vi "Flatten Value.vi"(8 "Error In":errorcluster, 11 "Path Array In":refnum<class "1D Path.lvclass">) -> (0 "Error Out":errorcluster, 1 "Value":string, 3 "Path Array Out":refnum<class "1D Path.lvclass">)   [LabVIEW 2017, in "Tree API.lvlib" / "1D Path.lvclass"]
uses:
  1D Path.lvclass
  Tree Manager/Tree.lvclass
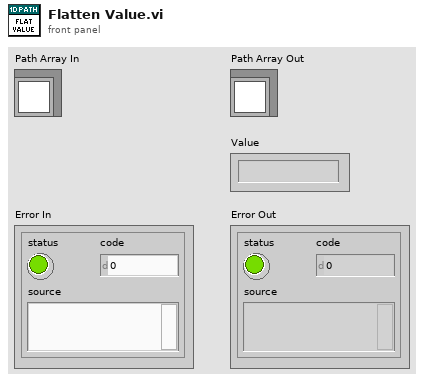
[diagram p1: front panel]
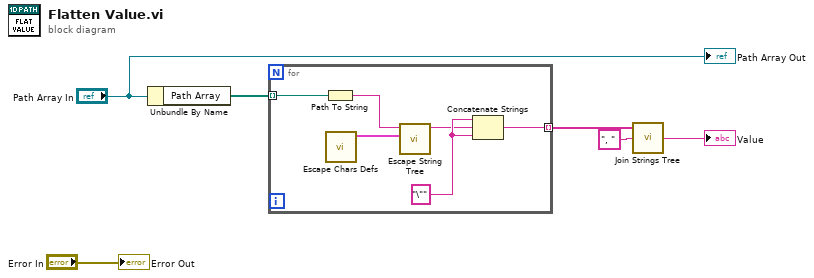
[diagram p0: block diagram]
diagram:
  n1 = Unbundle By Name("Path Array In") -> ("Path Array"=w6:path[])
  n2 = for {
    tunnel: w6 -> [w12] mode=indexing
    tunnel: [w10] -> w5 mode=indexing
    w11 = "\"" ("string")
    n3 = Path To String(path=w12) -> (string=w8:string)
    n4 = call "Escape Chars Defs.vi"() -> ("Escapes"=w9:cluster{"String":string, "Escape":string}[])  [unwired: 11 in]
    n5 = call "Escape String Tree.vi"("Escapes"=w9, "String In"=w8) -> ("String Out"=w7:string)  [unwired: 9 in]
    n6 = Concatenate Strings(w11, w7, w11) -> (w10:string)
  }
  n7 = call "Join Strings Tree.vi"("Separator (,)"=", ", "Strings In"=w5) -> ("String"=→"Value":string)  [unwired: 1 in]
  "Path Array Out" <- "Path Array In"
  "Error Out" <- "Error In"
